vi "model.vi"(0 "Joints.urdf":string, 2 "Links.urdf":string, 3 "Name":string) -> (4 "urdf out":string)   [LabVIEW 2012]
panel:
  # "transmission and gazebo"
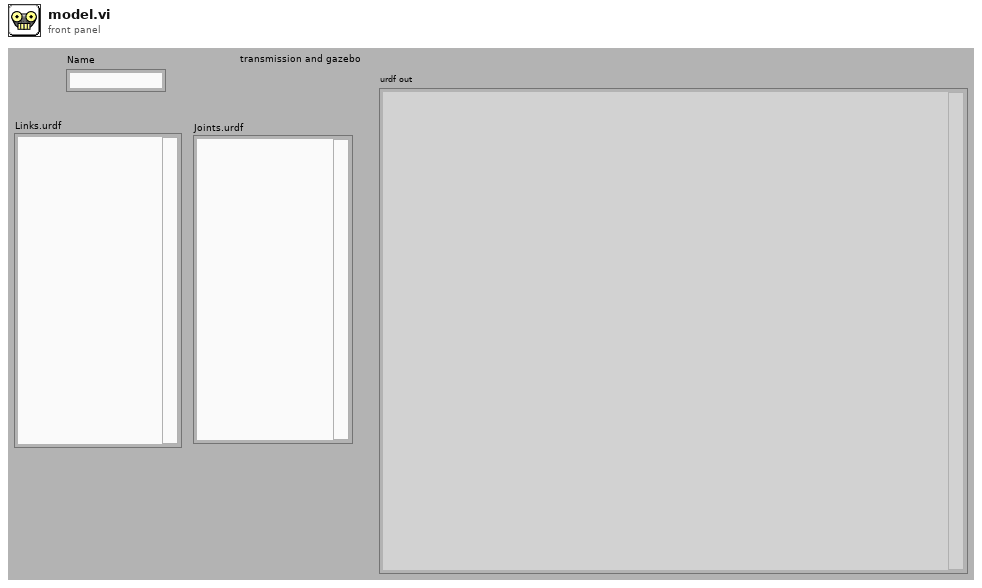
[diagram p1: front panel]
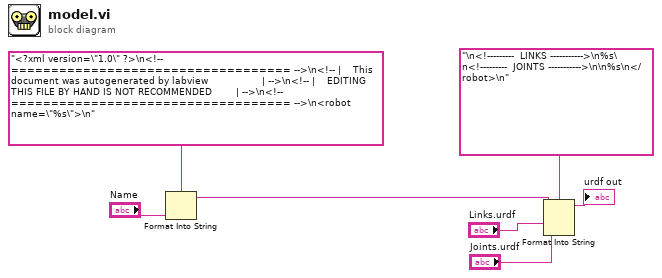
[diagram p0: block diagram]
diagram:
  n1 = Format Into String(format string="<?xml version=\"1.0\" ?>\n<!-- =================================== -->\n<!-- |    This document was autogenerated by labview                  | -->\n<!-- |    EDITING THIS FILE BY HAND IS NOT RECOMMENDED        | -->\n<!-- =================================== -->\n<robot name=\"%s\">\n", "Name") -> (resulting string=w3:string)  [unwired: 2 in, 1 out]
  n2 = Format Into String(format string="\n<!---------  LINKS ----------->\n%s\n<!---------  JOINTS ----------->\n\n%s\n</robot>\n", initial string=w3, "Links.urdf", "Joints.urdf") -> (resulting string=→"urdf out":string)  [unwired: 1 in, 1 out]
